vi "Shift State WrapAround.vi"(6 "Lower bound":i32, 7 "Upper bound":i32, 9 "Decrement":bool, 10 "Increment":bool, 11 "State in":i32) -> (3 "State out":i32)   [LabVIEW 2014]
doc: "Shifts a state up or down by 1.\nWraps around the ends - moving one past the top will wrap to the bottom, and vice versa.\nUsed in the operation of the clapper."
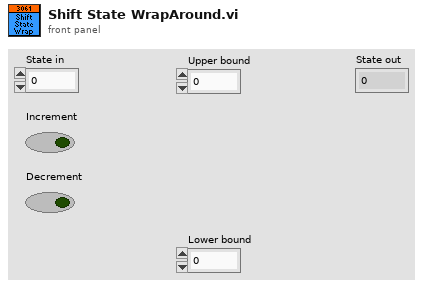
[diagram p1: front panel]
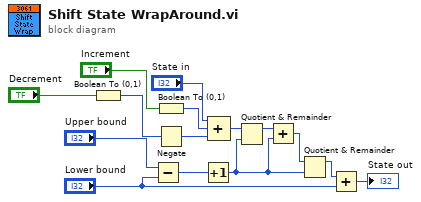
[diagram p0: block diagram]
diagram:
  n1 = Boolean To (0,1)(Boolean="Decrement") -> (0, 1=w13:i16)
  n2 = Subtract(x="Upper bound", y="Lower bound") -> (x-y=w7:i32)
  n3 = Boolean To (0,1)(Boolean="Increment") -> (0, 1=w11:i16)
  n4 = Negate(x=w13) -> (-x=w10:i16)
  n5 = Increment(x=w7) -> (x+1=w4:i32)
  n6 = Compound Arithmetic op=ADD("State in", w11, w10) -> (w8:i32)
  n7 = Quotient & Remainder(x=w8, y=w4) -> (x-y*floor(x/y)=w6:i32)  [unwired: 1 out]
  n8 = Add(x=w6, y=w4) -> (x+y=w5:i32)
  n9 = Quotient & Remainder(x=w5, y=w4) -> (x-y*floor(x/y)=w3:i32)  [unwired: 1 out]
  n10 = Add(x=w3, y="Lower bound") -> (x+y=→"State out":i32)
